vi "GettAllStuffsFromDAQmxTask.vi"(11 "task out":refnum<k21>) -> (3 "output cluster":T2={"Channels"=["PXI1Slot7/ao0", "PXI1Slot7/ao1"], "DeviceIsSimulated"=[FALSE], "ProductCategory"=[14649], "ProductType"=["PXI-4461"], "ProductNum"=[10400], "DevSerialNum"=[14550922], "Accessory.ProductTypes"=[[""]], "Accessory.ProductNums"=[[0]], "Accessory.SerialNums"=[[0]], "CarrierSerialNum"=[0], "Name"="", "NumChans"=2, "NumDevices"=1, "Done"=FALSE})   [LabVIEW 2016]
uses:
  <resource>/objmgr/daqmx.rc
panel:
  out "MNK":T1(array[cluster])=[{"Channels"=["PXI1Slot2/ai0", "PXI1Slot2/ai1"], "DeviceIsSimulated"=[FALSE], "ProductCategory"=[14649], "ProductType"=["PXI-4461"], "ProductNum"=[29299], "DevSerialNum"=[20525895], "Accessory.ProductTypes"=[[""]], "Accessory.ProductNums"=[[0]], "Accessory.SerialNums"=[[0]], "CarrierSerialNum"=[0], "Name"="", "NumChans"=2, "NumDevices"=1, "Done"=FALSE}, {"Channels"=["PXI1Slot3/ai0", "PXI1Slot3/ai1"], "DeviceIsSimulated"=[FALSE], "ProductCategory"=[14649], "ProductType"=["PXI-4461"], "ProductNum"=[29299], "DevSerialNum"=[21344870], "Accessory.ProductTypes"=[[""]], "Accessory.ProductNums"=[[0]], "Accessory.SerialNums"=[[0]], "CarrierSerialNum"=[0], "Name"="", "NumChans"=2, "NumDevices"=1, "Done"=FALSE}, {"Channels"=["PXI1Slot5/ai0", "PXI1Slot5/ai1"], "DeviceIsSimulated"=[FALSE], "ProductCategory"=[14649], "ProductType"=["PXI-4461"], "ProductNum"=[29299], "DevSerialNum"=[20763706], "Accessory.ProductTypes"=[[""]], "Accessory.ProductNums"=[[0]], "Accessory.SerialNums"=[[0]], "CarrierSerialNum"=[0], "Name"="", "NumChans"=2, "NumDevices"=1, "Done"=FALSE}, {"Channels"=["PXI1Slot7/ai0", "PXI1Slot7/ai1"], "DeviceIsSimulated"=[FALSE], "ProductCategory"=[14649], "ProductType"=["PXI-4461"], "ProductNum"=[10400], "DevSerialNum"=[14550922], "Accessory.ProductTypes"=[[""]], "Accessory.ProductNums"=[[0]], "Accessory.SerialNums"=[[0]], "CarrierSerialNum"=[0], "Name"="", "NumChans"=2, "NumDevices"=1, "Done"=FALSE}, {"Channels"=["PXI1Slot2/ao0", "PXI1Slot2/ao1"], "DeviceIsSimulated"=[FALSE], "ProductCategory"=[14649], "ProductType"=["PXI-4461"], "ProductNum"=[29299], "DevSerialNum"=[20525895], "Accessory.ProductTypes"=[[""]], "Accessory.ProductNums"=[[0]], "Accessory.SerialNums"=[[0]], "CarrierSerialNum"=[0], "Name"="", "NumChans"=2, "NumDevices"=1, "Done"=FALSE}, {"Channels"=["PXI1Slot3/ao0", "PXI1Slot3/ao1"], "DeviceIsSimulated"=[FALSE], "ProductCategory"=[14649], "ProductType"=["PXI-4461"], "ProductNum"=[29299], "DevSerialNum"=[21344870], "Accessory.ProductTypes"=[[""]], "Accessory.ProductNums"=[[0]], "Accessory.SerialNums"=[[0]], "CarrierSerialNum"=[0], "Name"="", "NumChans"=2, "NumDevices"=1, "Done"=FALSE}, {"Channels"=["PXI1Slot5/ao0", "PXI1Slot5/ao1"], "DeviceIsSimulated"=[FALSE], "ProductCategory"=[14649], "ProductType"=["PXI-4461"], "ProductNum"=[29299], "DevSerialNum"=[20763706], "Accessory.ProductTypes"=[[""]], "Accessory.ProductNums"=[[0]], "Accessory.SerialNums"=[[0]], "CarrierSerialNum"=[0], "Name"="", "NumChans"=2, "NumDevices"=1, "Done"=FALSE}, {"Channels"=["PXI1Slot7/ao0", "PXI1Slot7/ao1"], "DeviceIsSimulated"=[FALSE], "ProductCategory"=[14649], "ProductType"=["PXI-4461"], "ProductNum"=[10400], "DevSerialNum"=[14550922], "Accessory.ProductTypes"=[[""]], "Accessory.ProductNums"=[[0]], "Accessory.SerialNums"=[[0]], "CarrierSerialNum"=[0], "Name"="", "NumChans"=2, "NumDevices"=1, "Done"=FALSE}]
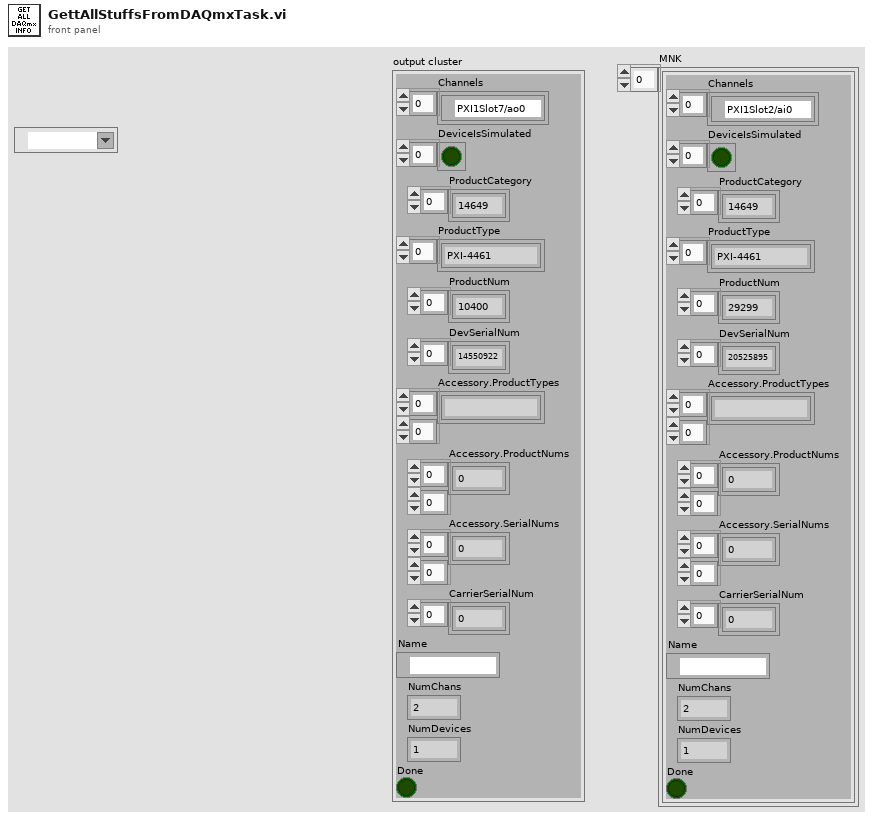
[diagram p1: front panel]
types:
  T1 = cluster{"Channels":refnum<k21>[], "DeviceIsSimulated":bool[], "ProductCategory":i32[], "ProductType":string[], "ProductNum":u32[], "DevSerialNum":u32[], "Accessory.ProductTypes":string[][], "Accessory.ProductNums":u32[][], "Accessory.SerialNums":u32[][], "CarrierSerialNum":u32[], "Name":refnum<k21>, "NumChans":u32, "NumDevices":u32, "Done":bool}[]
  T2 = cluster{"Channels":refnum<k21>[], "DeviceIsSimulated":bool[], "ProductCategory":i32[], "ProductType":string[], "ProductNum":u32[], "DevSerialNum":u32[], "Accessory.ProductTypes":string[][], "Accessory.ProductNums":u32[][], "Accessory.SerialNums":u32[][], "CarrierSerialNum":u32[], "Name":refnum<k21>, "NumChans":u32, "NumDevices":u32, "Done":bool}
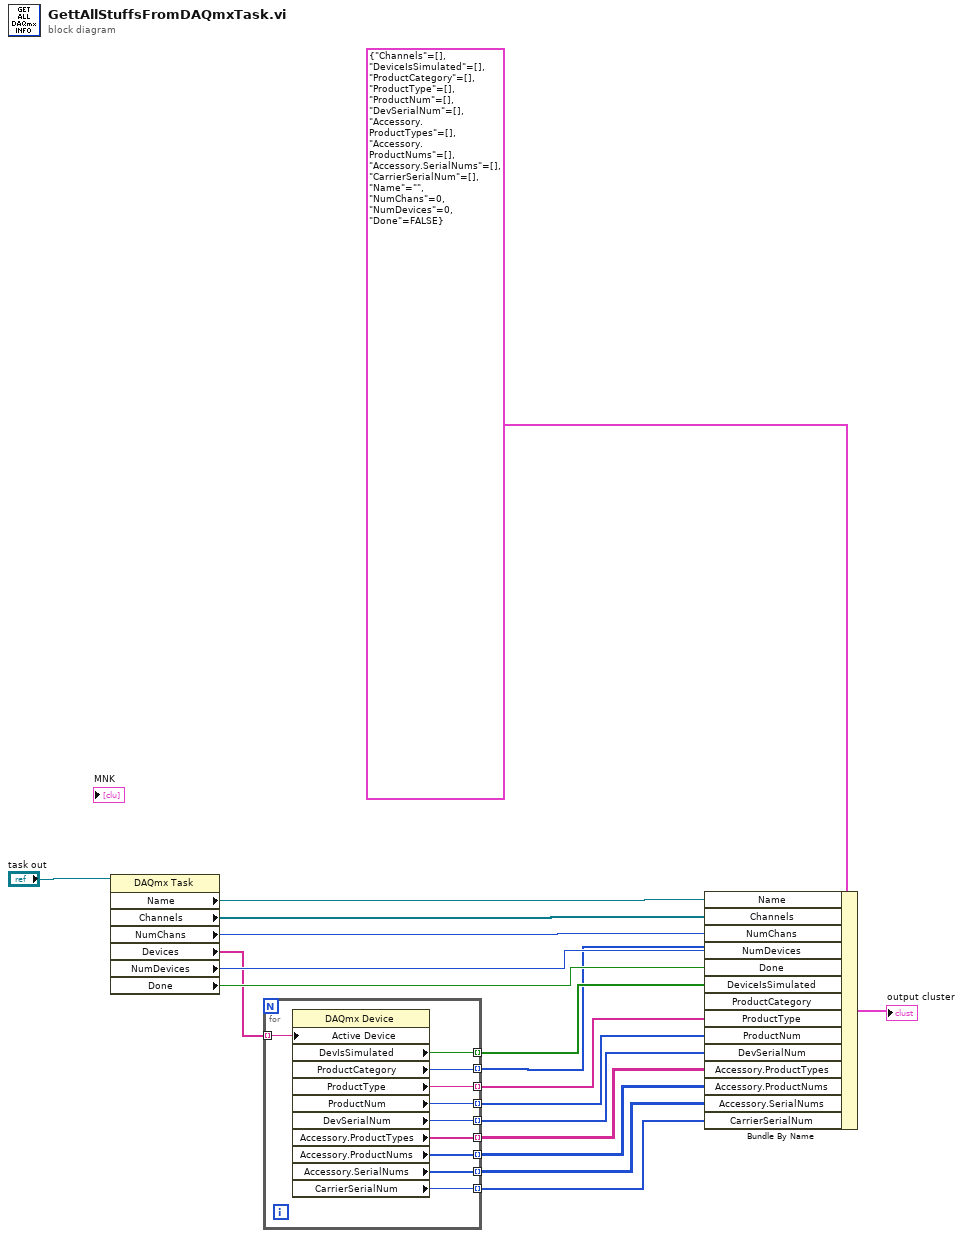
[diagram p0: block diagram]
diagram:
  n1 = property class="DAQmx Task"(reference="task out") -> ("Name"=w18:refnum<k21>, "Channels"=w17:refnum<k21>[], "NumChans"=w16:u32, "Devices"=w2:tag[], "NumDevices"=w15:u32, "Done"=w14:bool)  [unwired: 1 in, 2 out]
  n2 = for {
    tunnel: w2 -> [w28] mode=indexing
    tunnel: [w27] -> w13 mode=indexing
    tunnel: [w26] -> w12 mode=indexing
    tunnel: [w25] -> w11 mode=indexing
    tunnel: [w24] -> w10 mode=indexing
    tunnel: [w23] -> w9 mode=indexing
    tunnel: [w22] -> w8 mode=indexing
    tunnel: [w21] -> w7 mode=indexing
    tunnel: [w20] -> w6 mode=indexing
    tunnel: [w19] -> w5 mode=indexing
    n3 = property class="DAQmx Device"("Active Device"=w28) -> ("DevIsSimulated"=w27:bool, "ProductCategory"=w26:i32, "ProductType"=w25:string, "ProductNum"=w24:u32, "DevSerialNum"=w23:u32, "Accessory.ProductTypes"=w22:string[], "Accessory.ProductNums"=w21:u32[], "Accessory.SerialNums"=w20:u32[], "CarrierSerialNum"=w19:u32)  [unwired: 2 in, 2 out]
  }
  n4 = Bundle By Name(cluster=T2 {"Channels"=[], "DeviceIsSimulated"=[], "ProductCategory"=[], "ProductType"=[], "ProductNum"=[], "DevSerialNum"=[], "Accessory.ProductTypes"=[], "Accessory.ProductNums"=[], "Accessory.SerialNums"=[], "CarrierSerialNum"=[], "Name"="", "NumChans"=0, "NumDevices"=0, "Done"=FALSE}, "Name"=w18, "Channels"=w17, "NumChans"=w16, "NumDevices"=w15, "Done"=w14, "DeviceIsSimulated"=w13, "ProductCategory"=w12, "ProductType"=w11, "ProductNum"=w10, "DevSerialNum"=w9, "Accessory.ProductTypes"=w8, "Accessory.ProductNums"=w7, "Accessory.SerialNums"=w6, "CarrierSerialNum"=w5) -> (→"output cluster":T2)
